vi "API_Stop Tool Module.vi"(8 "error in (no error)":errorcluster) -> (0 "error out":errorcluster)   [LabVIEW 2015, in "Tool Module.lvlib"]
doc: "Send the Stop Module request to the Tool Module Main.vi. This vi does not wait for Main to close. You can wait on the \"Tool Module Broadcast Events.Module Did Stop\" user event to see if the Tool Module actually stopped."
uses:
  Tool Module.lvlib
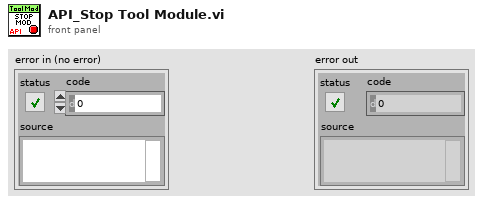
[diagram p1: front panel]
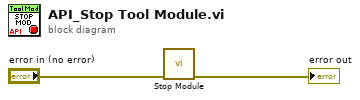
[diagram p0: block diagram]
diagram:
  n1 = call "Stop Module.vi"("error in (no error)"="error in (no error)") -> ("error out"=→"error out":errorcluster)  [unwired: 10 in]
